vi "Handle Errors.vi"(6 "Prompt? (T)":bool=TRUE, 8 "error in (no error)":errorcluster) -> (0 "error out":errorcluster)   [LabVIEW 2017, in "TSC Error.lvlib"]
doc: "This VI will handle errors in the application and is to be used after any loop where errors may exist. \n\nInputs:\n-error in (no error)\n-Prompt? (T) [Boolean] - this will prompt the user if set to TRUE; some cases, it is desired to not prompt the user\n\nOutputs:\n-error out\n__________________________________\n<b>Code Developed By:</b>\nDaniel Coons\nTechnology Service Corporation\n1983 S Liberty Drive\nBloomington, IN 47403\nPhone: 812 558-7100\ndaniel.coons@tsc.com\nwww.tsc.com\n\n<b>Date Created:</b> 11 AUG 2014\n<b>Date Updated:</b>"
uses:
  TSC Error.lvlib
  _Messages/ERROR_Write/ERROR_Write.lvclass
  _Messages/ERROR_Prompt/ERROR_Prompt.lvclass
  _Messages/Error/Error.lvclass
  C:/Development/Reuse-libraries/Error/_Messages/Error/Error.lvclass
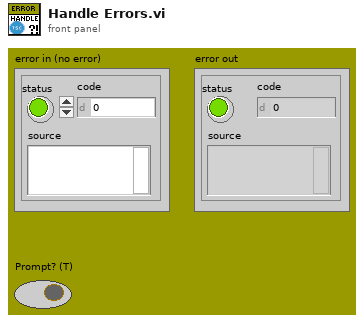
[diagram p1: front panel]
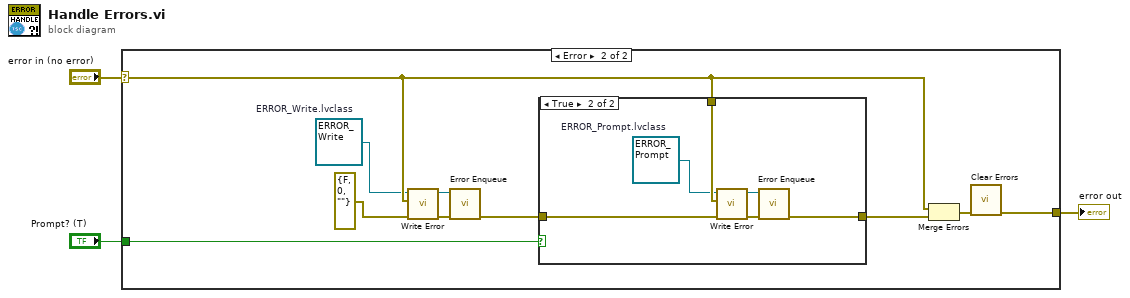
[diagram p0: block diagram]
diagram:
  n1 = case shown="Error" "error in (no error)" {
    selector: "error in (no error)" -> [w4 w12]
    tunnel: [w4 w10] -> w2
    tunnel: "Prompt? (T)" -> [_ w5]
    frame No Error {
    }
    frame Error {
      w7 = refnum<class "ERROR_Write.lvclass"> refnum  # ERROR_Write.lvclass
      n2 = call "Write Error.vi"("error in (no error)"=errorcluster {"status"=FALSE, "code"=0, "source"=""}, "Error"=w12, "Error in"=w7) -> ("error out"=w14:errorcluster, "Error out"=w9:refnum<class "ERROR_Write.lvclass">)  [unwired: 7 in]
      n3 = call "Error Enqueue.vi"("error in"=w14, "Error Message in"=w9) -> ("error out"=w8:errorcluster)  [unwired: 8 in, 1 out]
      n4 = case shown="True" w5 {
        tunnel: w12 -> [_ w20]
        tunnel: [w15 w19] -> w11
        tunnel: w8 -> [w15 w16]
        frame False {
        }
        frame True {
          w17 = refnum<class "ERROR_Prompt.lvclass"> refnum  # ERROR_Prompt.lvclass
          n5 = call "Write Error.vi"("error in (no error)"=w16, "Error"=w20, "Error in"=w17) -> ("error out"=w21:errorcluster, "Error out"=w18:refnum<class "ERROR_Prompt.lvclass">)  [unwired: 7 in]
          n6 = call "Error Enqueue.vi"("error in"=w21, "Error Message in"=w18) -> ("error out"=w19:errorcluster)  [unwired: 8 in, 1 out]
        }
      }
      n7 = Merge Errors(w12, w11) -> (w13:errorcluster)
      n8 = call <vilib>:"Clear Errors.vi"("error in (no error)"=w13) -> ("error out"=w10:errorcluster)  [unwired: 5 in, 1 out]
    }
  }
  "error out" <- w2
